vi "2DGaussianDemo.vi"(3 "output control":T1, 4 "data":variant, 5 "X":dbl[](array[numeric]), 6 "Coefficients":dbl[](array[numeric])) -> (0 "error out":errorcluster, 1 "f'(X,a)":dbl[][](array[numeric]), 2 "f(X,a)":dbl[](array[numeric]))   [LabVIEW 2015]
uses:
  <vilib>/gmath/NumericalOptimization/LM_output select.ctl
  <vilib>/gmath/NI_Gmath.lvlib
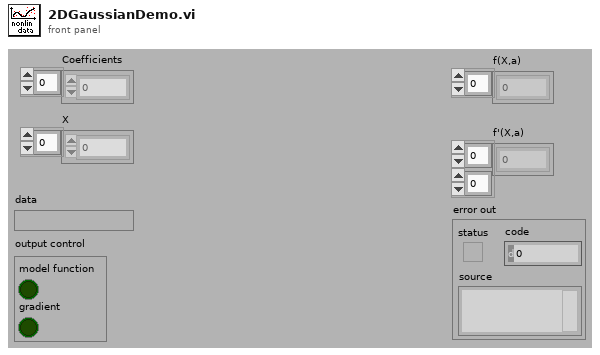
[diagram p1: front panel]
types:
  T1 = typedef "NI_Gmath.lvlib/LM_output select.ctl" = cluster{"model function":bool, "gradient":bool}
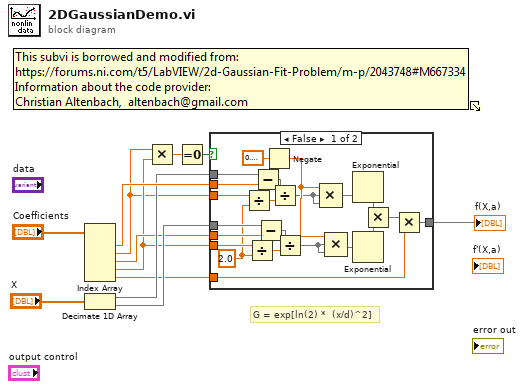
[diagram p0: block diagram]
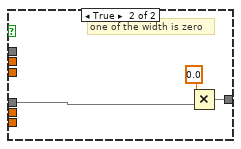
[diagram p2: hidden frame]
diagram:
  # "G = exp[ln(2) *  (x/d)^2]"
  n1 = Index Array(array="Coefficients") -> (element #1=w12:dbl, element #2=w4:dbl, element #3=w9:dbl, element #4=w8:dbl, element #5=w3:dbl)  [unwired: 5 in]
  n2 = Decimate 1D Array("X") -> (w11:dbl[], w10:dbl[])
  n3 = Multiply(x=w4, y=w8) -> (x*y=w7:dbl)
  n4 = Equal To 0?(x=w7) -> (x = 0?=w6:bool)
  n5 = case shown="False" w6 {
    tunnel: w12 -> [w34 _]
    tunnel: w11 -> [w33 _]
    tunnel: w4 -> [w32 _]
    tunnel: w10 -> [w31 w35]
    tunnel: w9 -> [w30 _]
    tunnel: w8 -> [w27 _]
    tunnel: [w24 w36] -> w1
    tunnel: w3 -> [w23 _]
    frame False {
      w25 = 2.0 ("y")
      n6 = Divide(x=w32, y=w25) -> (x/y=w28:dbl)
      n7 = Divide(x=w27, y=w25) -> (x/y=w26:dbl)
      n8 = Subtract(x=w33, y=w34) -> (x-y=w18:dbl[])
      n9 = Subtract(x=w31, y=w30) -> (x-y=w17:dbl[])
      n10 = Negate(x=0.6931471805599453) -> (-x=w21:dbl)
      n11 = Divide(x=w18, y=w28) -> (x/y=w19:dbl[])
      n12 = Divide(x=w17, y=w26) -> (x/y=w16:dbl[])
      n13 = Compound Arithmetic op=MULTIPLY(w21, w19, w19) -> (w20:dbl[])
      n14 = Compound Arithmetic op=MULTIPLY(w21, w16, w16) -> (w15:dbl[])
      n15 = Exponential(1:w20) -> (0:w13:dbl[])
      n16 = Exponential(1:w15) -> (0:w14:dbl[])
      n17 = Multiply(x=w13, y=w14) -> (x*y=w29:dbl[])
      n18 = Multiply(x=w29, y=w23) -> (x*y=w24:dbl[])
    }
    frame True {
      # "one of the width is zero"
      n19 = Multiply(x=0.0, y=w35) -> (x*y=w36:dbl[])
    }
  }
  "f(X,a)" <- w1
